vi "Write session info.vi"(8 "error in (no error)":errorcluster, 10 "session info":T1 {"last get" format="%x"; "last set" format="%x"}, 11 "VD-LV-LiteVNA in":refnum<class "VD-LV-LiteVNA.lvclass">) -> (0 "error out":errorcluster, 3 "VD-LV-LiteVNA out":refnum<class "VD-LV-LiteVNA.lvclass">)   [LabVIEW 2020, in "VD-LV-LiteVNA.lvclass"]
uses:
  VD-LV-LiteVNA.lvclass
  VD-session_info.ctl
  hardware-protocol/serial/HP-S-data.ctl
  VD-LV-LiteVNA.lvclass/VD-LV-LiteVNA.ctl
  hardware-protocol/serial/HP-S-Serial.lvclass
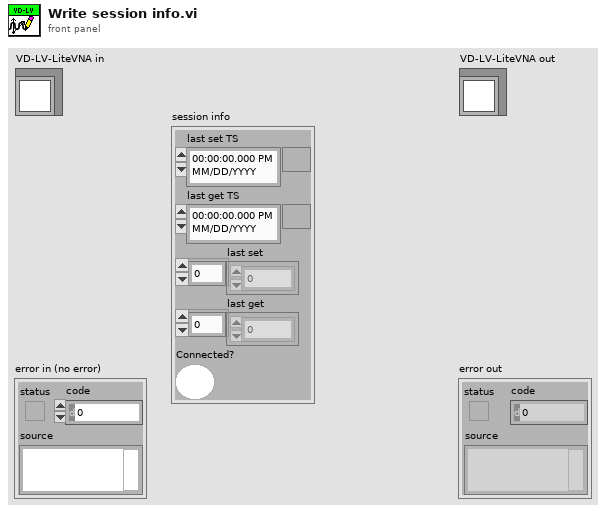
[diagram p1: front panel]
types:
  T1 = typedef "VD-LV-LiteVNA.lvclass/VD-session_info.ctl" = cluster{"last set TS":timestamp, "last get TS":timestamp, "last set":T2, "last get":T2, "Connected?":bool}
  T2 = typedef "HP-S-Serial.lvclass/HP-S-data.ctl" = u8[]
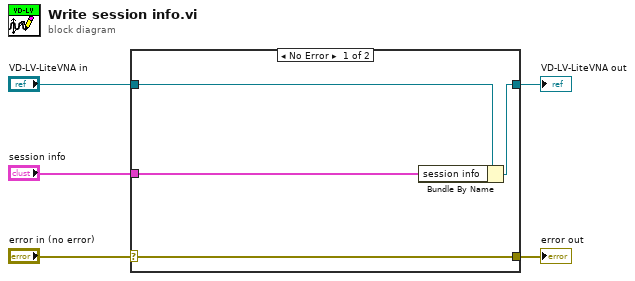
[diagram p0: block diagram]
diagram:
  n1 = case shown="No Error" "error in (no error)" {
    selector: "error in (no error)" -> [w9 w10]
    tunnel: [w9 w10] -> w4
    tunnel: [w7 w11] -> w2
    tunnel: "VD-LV-LiteVNA in" -> [w8 w11]
    tunnel: "session info" -> [w6 _]
    frame No Error {
      n2 = Bundle By Name(cluster=w8, "session info"=w6) -> (w7:refnum<class "VD-LV-LiteVNA.lvclass">)
    }
    frame Error {
    }
  }
  "error out" <- w4
  "VD-LV-LiteVNA out" <- w2
